vi "Simple_LV2.vi"(0 "Data_In":dbl format="%#_13g", 11 "Error_In":errorcluster, 13 "Operation":T1=enum."Read") -> (4 "Data_Out":dbl format="%#_13g", 15 "Error_Out":errorcluster)   [LabVIEW 2023]
doc: "This a simply LV2 which can be write and read accross VIs"
uses:
  Type_Def/Operation_Simple_LV2.ctl
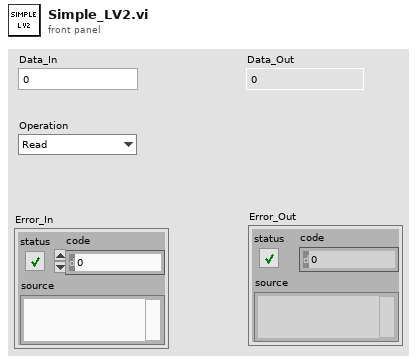
[diagram p1: front panel]
types:
  T1 = typedef "Operation_Simple_LV2.ctl" = enum16{"Write", "Read"}
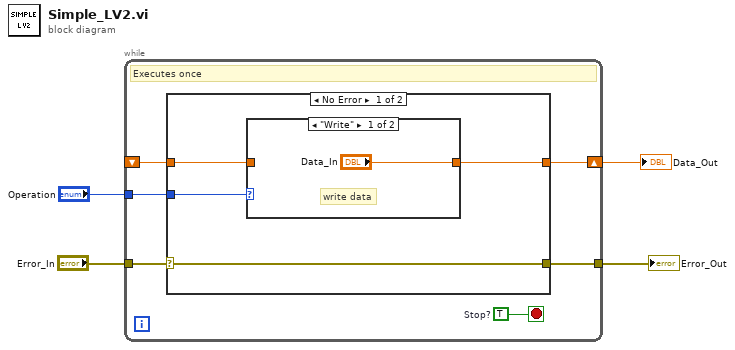
[diagram p0: block diagram]
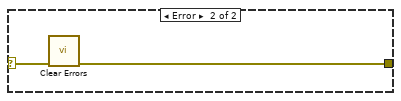
[diagram p3: hidden frame]
diagram:
  n1 = while {
    shift-right: [w10] -> w4
    shift-left: _ -> [w9]
    tunnel: "Operation" -> [w8]
    tunnel: "Error_In" -> [w7]
    tunnel: [w5] -> w1
    stop <- w6 stop-if-true
    w6 = TRUE  # Stop?
    # "Executes once"
    n2 = case shown="No Error" w7 {
      selector: w7 -> [w11 w18]
      tunnel: [w14 _] -> w10
      tunnel: w9 -> [w13 _]
      tunnel: w8 -> [w12 _]
      tunnel: [w11 w17] -> w5
      frame No Error {
        n3 = case shown="\"Write\"" w12 {
          tunnel: ["Data_In" w16] -> w14
          tunnel: w13 -> [_ w16]
          frame "Write" {
            # "write data"
          }
          frame "Read" {
            # "Read data"
          }
        }
      }
      frame Error {
        n4 = call <vilib>:"Clear Errors.vi"("error in (no error)"=w18) -> ("error out"=w17:errorcluster)  [unwired: 5 in, 1 out]
      }
    }
  }
  "Error_Out" <- w1
  "Data_Out" <- w4
